vi "ErrorHandler.vi"(8 "error in (no error)":errorcluster) -> (0 "error out":errorcluster)   [LabVIEW 2017, in "Server.lvlib" / "ErrorLogger.lvlib"]
doc: "This VI calls the ErrorHandlerFGV. This VI is Reentrant to avoid coupling between loops. Only in case of error it will call the Non-Reentrant ErrorHandlerFGV to send the Error to the Error-Queue."
uses:
  ErrorLogger.lvlib
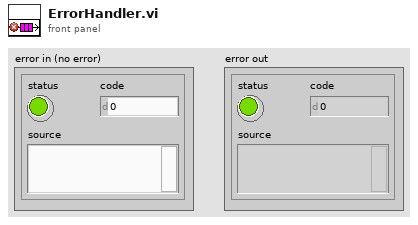
[diagram p1: front panel]
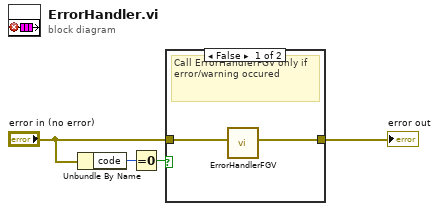
[diagram p0: block diagram]
diagram:
  n1 = Unbundle By Name("error in (no error)") -> ("code"=w2:i32)
  n2 = Equal To 0?(x=w2) -> (x = 0?=w1:bool)
  n3 = case shown="False" w1 {
    tunnel: [w6 w7] -> w4
    tunnel: "error in (no error)" -> [w5 w7]
    frame False {
      # "Call ErrorHandlerFGV only if error/warning occured"
      n4 = call "ErrorHandlerFGV.vi"("Error In"=w5) -> ("Error Out"=w6:errorcluster)  [unwired: 10 in]
    }
    frame True {
    }
  }
  "error out" <- w4
